vi "UI Initialize.vi"(8 "error in (no error)":errorcluster, 11 "UI Wizard in":refnum<class "UI Wizard.lvclass">) -> (0 "error out":errorcluster, 3 "UI Wizard out":refnum<class "UI Wizard.lvclass">)   [LabVIEW 2013, in "SET Project Editor.lvlib" / "UI Wizard.lvclass"]
uses:
  UI Wizard.lvclass
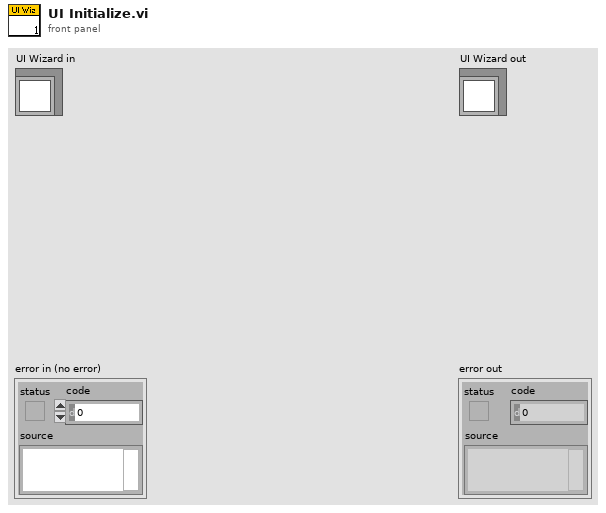
[diagram p1: front panel]
types:
  T1 = enum32{"Invalid", "Standard", "Closed", "Hidden", "Minimized", "Maximized"}
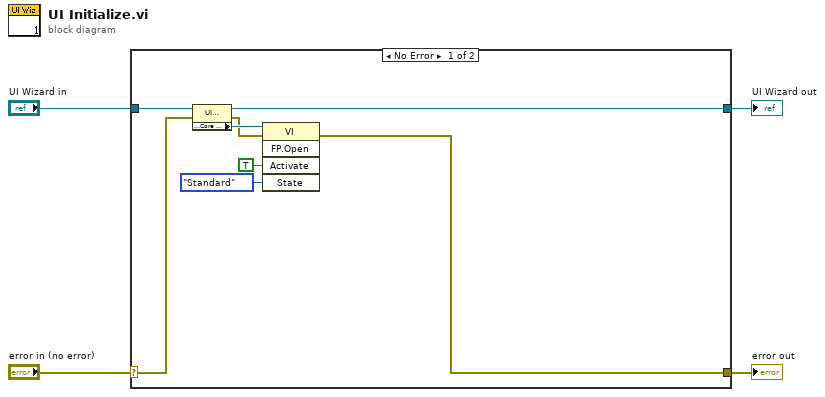
[diagram p0: block diagram]
diagram:
  n1 = case shown="No Error" "error in (no error)" {
    selector: "error in (no error)" -> [w6 w14]
    tunnel: [w5 w14] -> w3
    tunnel: [w7 w13] -> w1
    tunnel: "UI Wizard in" -> [w8 w13]
    frame No Error {
      n2 = property class="UI Wizard.lvclass"(reference=w8, error in=w6) -> (reference out=w7:refnum<class "UI Wizard.lvclass">, error out=w9:errorcluster, "Properties:Core VI Refnum"=w12:refnum<vi>)
      n3 = invoke class="VI" method="FP.Open"(reference=w12, error in=w9, "Activate"=TRUE ("Activate?"), "State"=T1."Standard") -> (error out=w5:errorcluster)  [unwired: 1 in, 4 out]
    }
    frame Error {
    }
  }
  "error out" <- w3
  "UI Wizard out" <- w1
